vi "Actor Core.vi"(8 "error in":errorcluster, 11 "CO2 Actor in":refnum<class "CO2 Actor.lvclass">) -> (0 "error out":errorcluster, 3 "Actor out":refnum<class "Actor.lvclass">)   [LabVIEW 2015, in "cRIO-Carbondioxide.lvlib" / "CO2-Actor.lvlib" / "CO2 Actor.lvclass"]
doc: "(<B>Filename</B>: Actor Framework.lvlib:Actor.lvclass:Actor Core.vi)\n\nReceives messages to the actor, reacts to them, and initiates any error handling that may shut the actor down.\n\nDescendant classes may override this VI to append parallel tasks for the actor to complete while it handles messages. Overrides use the Call Parent Method node."
uses:
  CO2 Actor.lvclass
  <vilib>/ActorFramework/Actor/Actor.lvclass
  CO2 Actor.lvclass/CO2 Actor.ctl
  Interlocks/Interlock Chain/Interlock Chain.lvclass
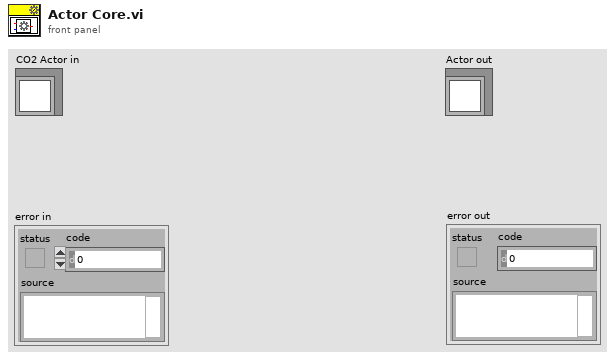
[diagram p1: front panel]
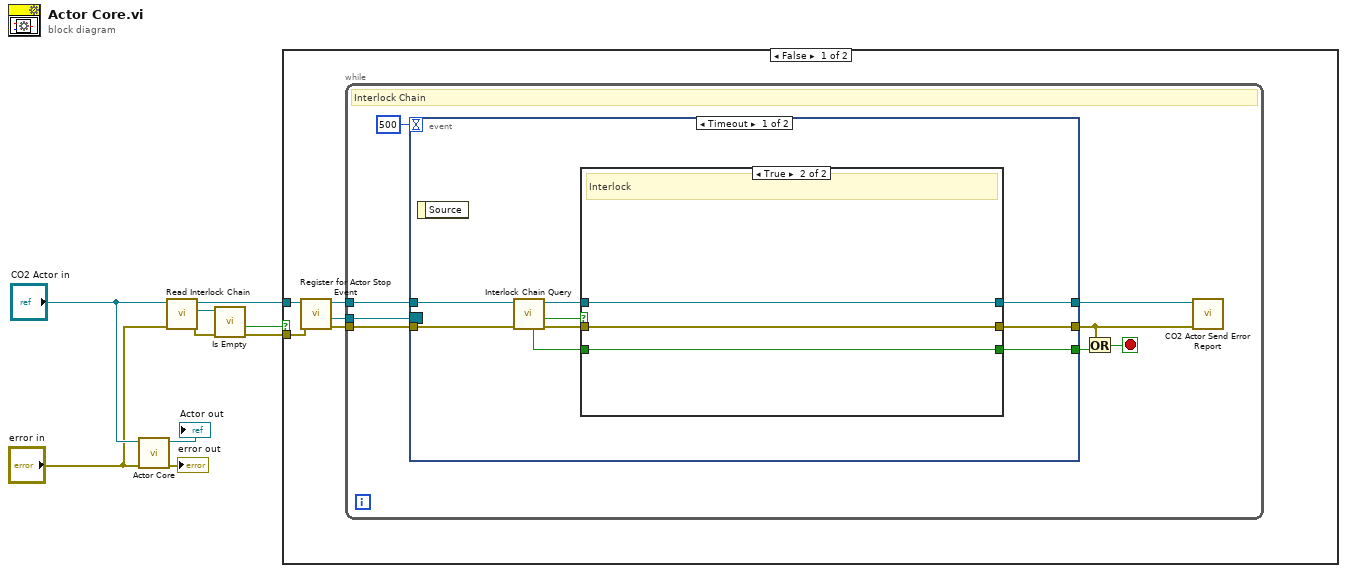
[diagram p0: block diagram]
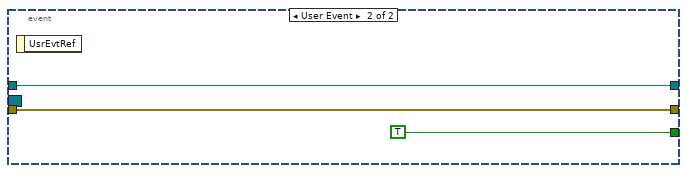
[diagram p3: hidden frame]
diagram:
  n1 = call-parent "Actor Core.vi"("error in"="error in", "Actor in"="CO2 Actor in") -> ("error out"=→"error out":errorcluster, "Actor out"=→"Actor out":refnum<class "Actor.lvclass">)  [unwired: 8 in]
  n2 = call "Read Interlock Chain.vi"("error in (no error)"="error in", "CO2 Actor in"="CO2 Actor in") -> ("error out"=w3:errorcluster, "Interlock Chain"=w4:refnum<class "Interlock Chain.lvclass">, "CO2 Actor out"=w7:refnum<class "CO2 Actor.lvclass">)  [unwired: 7 in]
  n3 = call "Is Empty.vi"("error in (no error)"=w3, "Interlock Chain in"=w4) -> ("error out"=w2:errorcluster, "Is Empty?"=w1:bool)  [unwired: 7 in, 1 out]
  n4 = case shown="False" w1 {
    tunnel: w7 -> [w11 _]
    tunnel: w2 -> [w10 _]
    frame False {
      n5 = call "Register for Actor Stop Event.vi"("error in (no error)"=w10, "CO2 Actor in"=w11) -> ("error out"=w13:errorcluster, "Event Registration Refnum"=w14:refnum<event-registration>, "CO2 Actor out"=w12:refnum<class "CO2 Actor.lvclass">)  [unwired: 7 in]
      n6 = while {
        tunnel: w14 -> [w21]
        tunnel: w13 -> [w20]
        tunnel: w12 -> [w19]
        stop <- w18 stop-if-true
        # "Interlock Chain"
        n7 = event shown="[0] Timeout" {
          selector: w21 -> [_ _]
          dyn-events: _ -> [_ _]
          timeout: 500 -> [_ _]
          tunnel: w20 -> [w30 w37]
          tunnel: w19 -> [w31 w38]
          tunnel: [w29 w37] -> w15
          tunnel: [w24 TRUE] -> w17
          tunnel: [w26 w38] -> w16
          event Timeout {
            n8 = event-data() -> ()  [unwired: 1 in, 1 out]
            n9 = call-dynamic "Interlock Chain Query.vi"("error in (no error)"=w30, "CO2 Actor in"=w31) -> ("error out"=w28:errorcluster, "Interlock out"=w25:bool, "CO2 Actor out"=w27:refnum<class "CO2 Actor.lvclass">, "Stop Self?"=w23:bool)  [unwired: 6 in]
            n10 = case shown="True" w25 {
              tunnel: w28 -> [w33 w36]
              tunnel: w27 -> [w32 w34]
              tunnel: [w33 w36] -> w29
              tunnel: [w32 w34] -> w26
              tunnel: [_ w35] -> w24
              tunnel: w23 -> [_ w35]
              frame False {
              }
              frame True {
                # "Interlock"
              }
            }
          }
          event User Event {
            n11 = event-data() -> ()  [unwired: 1 in, 1 out]
          }
        }
        n12 = Or(x=w15, y=w17) -> (x .or. y?=w18:bool)
        n13 = call-dynamic "CO2 Actor Send Error Report.vi"("Error From Sender"=w15, "CO2 Actor in"=w16) -> ()  [unwired: 9 in, 1 out]
      }
    }
    frame True {
      # "The chain is empty. Nothing to do here."
    }
  }
